vi "get NTP time.vi"(8 "error in (no error)":errorcluster, 11 "NTP server IP address":string="time.nist.gov") -> (0 "error out":errorcluster, 1 "NTP string":string, 3 "NTP time":timestamp)   [LabVIEW 2013]
uses:
  <vilib>/Utility/miscctls.llb/LVDateTimeRec.ctl
panel:
  # "get NTP time"
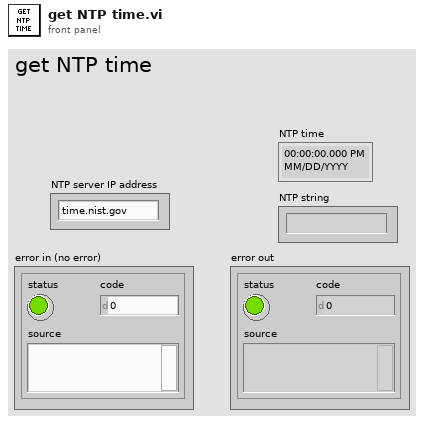
[diagram p1: front panel]
types:
  T1 = typedef "LVDateTimeRec.ctl" = cluster{"fractional second":dbl, "second":i32, "minute":i32, "hour":i32, "day of month":i32, "month":i32, "year":i32, "day of week":i32, "day of year":i32, "DST":i32}
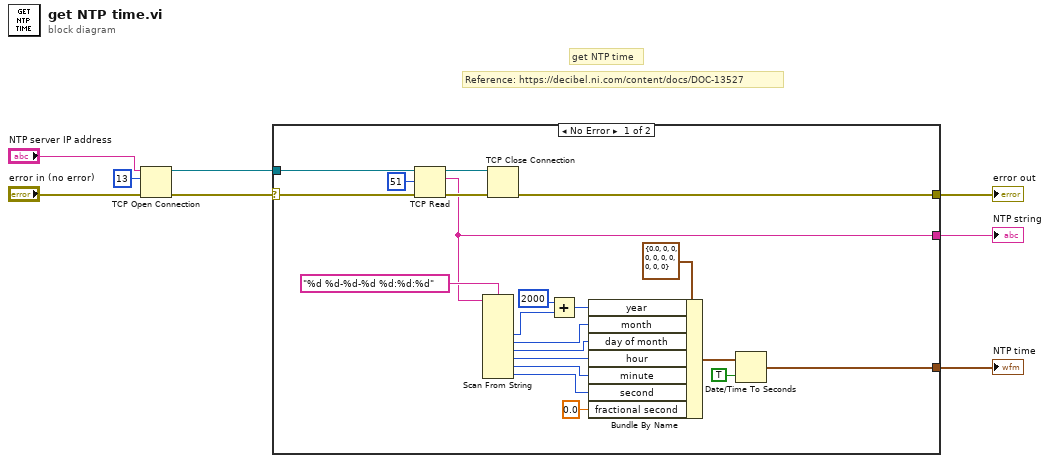
[diagram p0: block diagram]
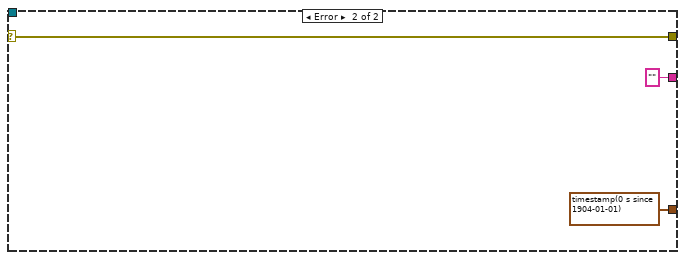
[diagram p2: hidden frame]
diagram:
  # "Reference: https://decibel.ni.com/content/docs/DOC-13527"
  # "get NTP time"
  n1 = TCP Open Connection(address="NTP server IP address", remote port or service name=u16 13 ("port"), error in (no error)="error in (no error)") -> (connection ID=w4:refnum<k5>, error out=w5:errorcluster)  [unwired: 2 in]
  n2 = case shown="No Error" w5 {
    selector: w5 -> [w13 w31]
    tunnel: w4 -> [w12 _]
    tunnel: [w11 timestamp(0 s since 1904-01-01) ("time stamp")] -> w3
    tunnel: [w10 w31] -> w2
    tunnel: [w9 "" ("data out")] -> w1
    frame No Error {
      n3 = TCP Read(connection ID=w12, bytes to read=51, error in (no error)=w13) -> (connection ID out=w28:refnum<k5>, data out=w9:string, error out=w27:errorcluster)  [unwired: 2 in]
      n4 = Scan From String(format string="%d %d-%d-%d %d:%d:%d", input string=w9) -> (output 2=w16:i32, output 3=w19:i32, output 4=w20:i32, output 5=w21:i32, output 6=w22:i32, output 7=w23:i32)  [unwired: 10 in, 3 out]
      n5 = TCP Close Connection(connection ID=w28, error in (no error)=w27) -> (error out=w10:errorcluster)  [unwired: 1 in, 1 out]
      n6 = Add(x=2000, y=w16) -> (x+y=w17:i32)
      n7 = Bundle By Name "Bundle By Name"(cluster=T1 {"fractional second"=0.0, "second"=0, "minute"=0, "hour"=0, "day of month"=0, "month"=0, "year"=0, "day of week"=0, "day of year"=0, "DST"=0} ("date time rec"), "year"=w17, "month"=w19, "day of month"=w20, "hour"=w21, "minute"=w22, "second"=w23, "fractional second"=0.0) -> (w24:T1)
      n8 = Date/Time To Seconds(1:TRUE ("is UTC (F)"), 2:w24) -> (0:w11:timestamp)
    }
    frame Error {
    }
  }
  "error out" <- w2
  "NTP time" <- w3
  "NTP string" <- w1
